vi "Table Initialize_2D.vi"(4 "행의 개수":u32, 5 "Table Ref":refnum<vi>, 6 "Value":string[][](array[string]), 7 "비활성화?":bool, 8 "에러 입력":errorcluster caption="에러 입력(에러 없음)", 9 "열해더 문자열":string[](array[string]), 10 "열의 개수":u32, 11 "최상단보기?":bool) -> (0 "에러 출력":errorcluster, 1 "Bottom":i32, 3 "Table Ref out":refnum<vi>)   [LabVIEW 2020]
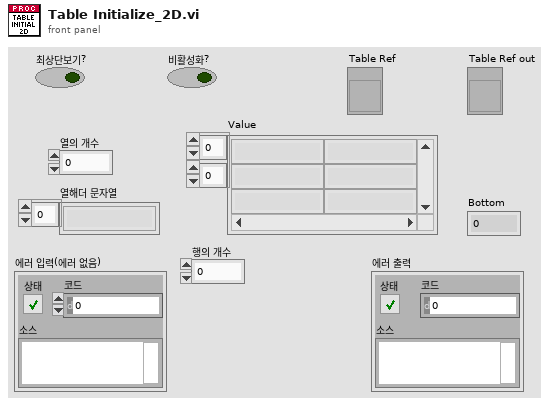
[diagram p1: front panel]
types:
  T1 = enum8{"Enabled", "Disabled", "Disabled and Grayed Out"}
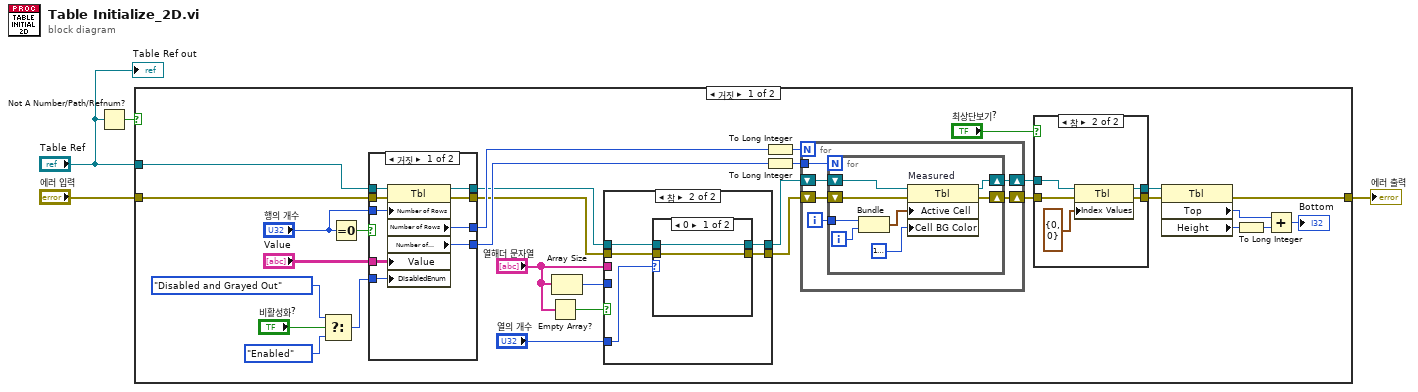
[diagram p0: block diagram]
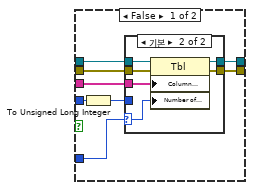
[diagram p2: hidden frame]
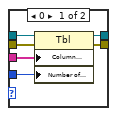
[diagram p3: hidden frame]
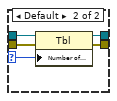
[diagram p4: hidden frame]
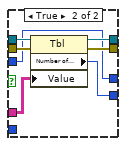
[diagram p6: hidden frame]
diagram:
  n1 = Not A Number/Path/Refnum?(number/path/refnum="Table Ref") -> (NaN/Path/Refnum?=w1:bool)
  n2 = case shown="거짓" w1 {
    tunnel: "에러 입력" -> [w35 w105]
    tunnel: "Table Ref" -> [w29 _]
    tunnel: [w23 w105] -> w3
    frame False {
      n3 = Select(t=T1."Disabled and Grayed Out" ("비활성화"), s="비활성화?", f=T1."Enabled" ("비활성화")) -> (s? t:f=w15:T1)
      n4 = Equal To 0?(x="행의 개수") -> (x = 0?=w27:bool)
      n5 = case shown="거짓" w27 {
        tunnel: w35 -> [w83 w90]
        tunnel: "Value" -> [w82 w89]
        tunnel: [w81 w88] -> w12
        tunnel: [w80 w87] -> w33
        tunnel: [w79 w86] -> w11
        tunnel: [w78 w84] -> w30
        tunnel: w29 -> [w77 w85]
        tunnel: "행의 개수" -> [w76 w84]
        tunnel: w15 -> [w75 _]
        frame False {
          n6 = property class="Tbl"(reference=w77, error in=w83, "Number of Rows"=w76, "Value"=w82, "DisabledEnum"=w75) -> (reference out=w79:refnum<vi>, error out=w81:errorcluster, "Number of Rows"=w78:u32, "Number of Columns"=w80:u32)
        }
        frame True {
          n7 = property class="Tbl"(reference=w85, error in=w90, "Value"=w89) -> (reference out=w86:refnum<vi>, error out=w88:errorcluster, "Number of Columns"=w87:u32)
        }
      }
      n8 = Empty Array?(array="열해더 문자열") -> (empty?=w10:bool)
      n9 = Array Size(array="열해더 문자열") -> (size(s)=w6:i32)
      n10 = case shown="참" w10 {
        tunnel: w12 -> [w43 w60]
        tunnel: [w42 w59] -> w8
        tunnel: [w41 w58] -> w9
        tunnel: w11 -> [w40 w57]
        tunnel: "열해더 문자열" -> [w39 _]
        tunnel: w6 -> [w38 _]
        tunnel: "열의 개수" -> [w36 w56]
        frame False {
          n11 = To Unsigned Long Integer(number=w38) -> (unsigned 32bit integer=w37:u32)
          n12 = case shown="기본" w36 {
            selector: w36 -> [_ w50]
            tunnel: w43 -> [w49 w55]
            tunnel: [w48 w54] -> w42
            tunnel: [w47 w53] -> w41
            tunnel: w40 -> [w46 w52]
            tunnel: w39 -> [w45 w51]
            tunnel: w37 -> [w44 _]
            frame 0 {
              n13 = property class="Tbl"(reference=w46, error in=w49, "Column Headers[]"=w45, "Number of Columns"=w44) -> (reference out=w47:refnum<vi>, error out=w48:errorcluster)
            }
            frame Default {
              n14 = property class="Tbl"(reference=w52, error in=w55, "Column Headers[]"=w51, "Number of Columns"=w50) -> (reference out=w53:refnum<vi>, error out=w54:errorcluster)
            }
          }
        }
        frame True {
          n15 = case shown="0" w56 {
            selector: w56 -> [_ w63]
            tunnel: w60 -> [w61 w67]
            tunnel: [w61 w66] -> w59
            tunnel: [w62 w65] -> w58
            tunnel: w57 -> [w62 w64]
            frame 0 {
            }
            frame Default {
              n16 = property class="Tbl"(reference=w64, error in=w67, "Number of Columns"=w63) -> (reference out=w65:refnum<vi>, error out=w66:errorcluster)
            }
          }
        }
      }
      n17 = To Long Integer(number=w30) -> (32bit integer=w32:i32)
      n18 = To Long Integer(number=w33) -> (32bit integer=w31:i32)
      n19 = for {
        N: w32 -> [_]
        shift-right: [w94] -> w26
        shift-left: w8 -> [w95]
        tunnel: w31 -> [w92]
        shift-right: [w91] -> w24
        shift-left: w9 -> [w96]
        i -> [w93]
        n20 = for {
          N: w92 -> [_]
          shift-right: [w102] -> w94
          shift-left: w95 -> [w103]
          tunnel: w93 -> [w101]
          shift-right: [w97] -> w91
          shift-left: w96 -> [w104]
          i -> [w100]
          n21 = Bundle(w101, w100) -> (w99:cluster{i32, i32})  [unwired: 1 in]
          n22 = property on="Measured" class="Tbl"(reference=w104, error in=w103, "Active Cell"=w99, "Cell BG Color"=u32 16777226) -> (reference out=w97:refnum<vi>, error out=w102:errorcluster)
        }
      }
      n23 = case shown="참" "최상단보기?" {
        tunnel: w26 -> [w69 w74]
        tunnel: [w69 w73] -> w14
        tunnel: w24 -> [w68 w72]
        tunnel: [w68 w70] -> w13
        frame False {
        }
        frame True {
          n24 = property class="Tbl"(reference=w72, error in=w74, "Index Values"=cluster{"Row":u32, "Column":u32} {"Row"=0, "Column"=0} ("인덱스 값")) -> (reference out=w70:refnum<vi>, error out=w73:errorcluster)
        }
      }
      n25 = property class="Tbl"(reference=w13, error in=w14) -> (error out=w23:errorcluster, "Top"=w21:i32, "Height"=w20:u32)  [unwired: 1 out]
      n26 = To Long Integer(number=w20) -> (32bit integer=w22:i32)
      n27 = Add(x=w21, y=w22) -> (x+y=→"Bottom":i32)
    }
    frame True {
    }
  }
  "에러 출력" <- w3
  "Table Ref out" <- "Table Ref"
